vi "data array refresh 500ms.vi"(8 "error in (no error)":errorcluster, 11 "queue out":refnum<queue>) -> (0 "error out":errorcluster, 3 "queue out 2":refnum<queue>)   [LabVIEW 2021]
panel:
  out "Array":dbl[][](array[numeric])
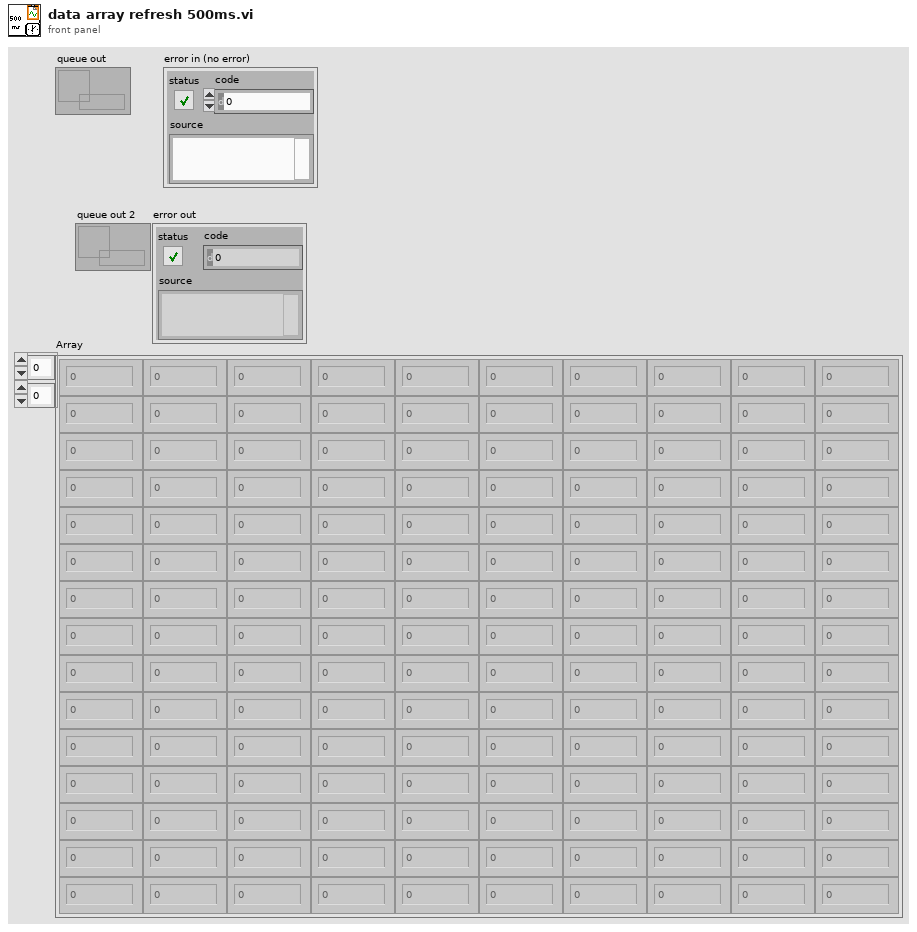
[diagram p1: front panel]
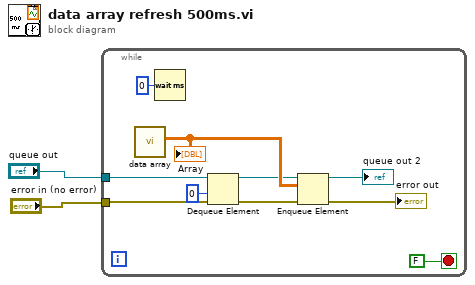
[diagram p0: block diagram]
diagram:
  n1 = while {
    tunnel: "error in (no error)" -> [w8]
    tunnel: "queue out" -> [w9]
    stop <- FALSE stop-if-true
    n2 = call "data array.vi"() -> ("Array"=w10:dbl[][])  [unwired: 11 in]
    "Array" <- w10
    n3 = Wait (ms)(milliseconds to wait=u32 0) -> ()  [unwired: 1 out]
    n4 = Dequeue Element(queue=w9, timeout in ms (-1)=0, error in (no error)=w8) -> (queue out=w7:refnum<queue>, error out=w6:errorcluster)  [unwired: 2 out]
    n5 = Enqueue Element(queue=w7, element=w10, error in (no error)=w6) -> (queue out=→"queue out 2":refnum<queue>, error out=→"error out":errorcluster)  [unwired: 1 in, 1 out]
  }
